vi "Athena Localization Data.vi"() -> ()   [LabVIEW 2009]
panel:
  in  "latitude":dbl
  in  "heading":dbl
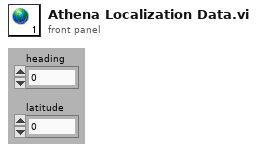
[diagram p1: front panel]
diagram:
